vi "cw_3_1.vi"() -> ()   [LabVIEW 2022 SP3]
panel:
  in  "M":i32
  out "Array":i32[][](array[numeric])
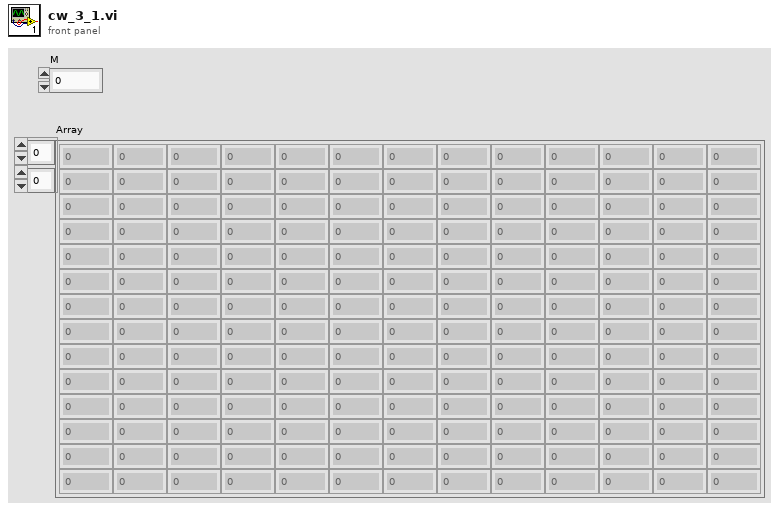
[diagram p1: front panel]
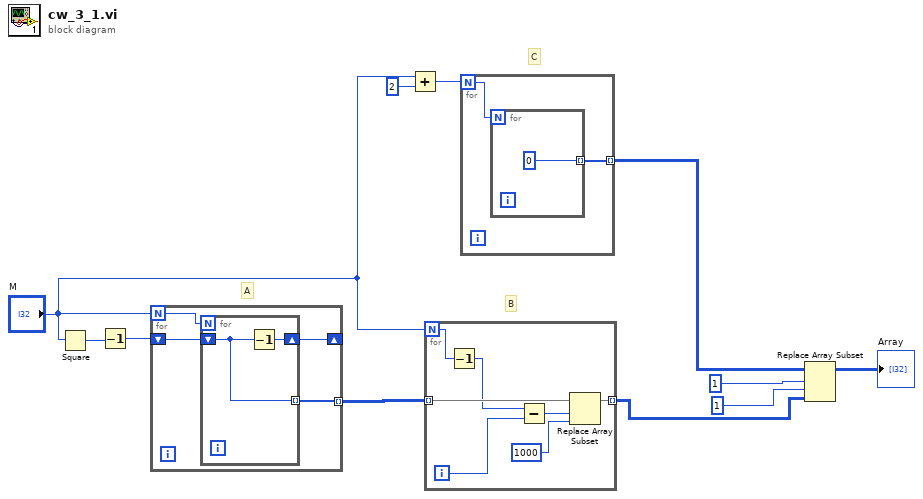
[diagram p0: block diagram]
diagram:
  # "C"
  # "B"
  # "A"
  n1 = Square(x="M") -> (x^2=w11:i32)
  n2 = Decrement(x=w11) -> (x-1=w10:i32)
  n3 = for {
    N: "M" -> [w14]
    tunnel: [w15] -> w9 mode=indexing
    shift-right: [w12] -> _
    shift-left: w10 -> [w13]
    n4 = for {
      N: w14 -> [_]
      tunnel: [w16] -> w15 mode=indexing
      shift-right: [w17] -> w12
      shift-left: w13 -> [w16]
      n5 = Decrement(x=w16) -> (x-1=w17:i32)
    }
  }
  n6 = Add(x="M", y=2) -> (x+y=w1:i32)
  n7 = for {
    N: "M" -> [w19]
    tunnel: w9 -> [w23] mode=indexing
    tunnel: [w22] -> w7 mode=indexing
    i -> [w20]
    n8 = Decrement(x=w19) -> (x-1=w18:i32)
    n9 = Subtract(x=w18, y=w20) -> (x-y=w21:i32)
    n10 = Replace Array Subset(array=w23, new element=1000 ("new element/subarray"), index=w21) -> (w22:i32[])
  }
  n11 = for {
    N: w1 -> [w26]
    tunnel: [w25] -> w8 mode=indexing
    n12 = for {
      N: w26 -> [_]
      tunnel: [0] -> w25 mode=indexing
    }
  }
  n13 = Replace Array Subset(array=w8, new element=w7, index (row)=1 ("disabled index (row)"), index (col)=1 ("disabled index (col)")) -> (→"Array":i32[][])
